vi "Construct Ring Strings Binding.vi"(10 "Ring Refnum":refnum<vi>) -> (0 "error out":errorcluster, 3 "RingStringsBinding":refnum<class "RingStringsBinding.lvclass">)   [LabVIEW 2019, in "RingStringsBinding.lvclass"]
doc: "<License>\nCopyright © 2017 Composed Systems, LLC | All rights reserved\nwww.composed.io\n\nAuthor: Ethan Stern <ethan.stern@composed.io>\n\nThis software is provided \"AS IS\" WITHOUT WARRANTIES, either express or implied, AND IS FOR EDUCATIONAL PURPOSES ONLY.\n</License>MVA Framework 1.0.4.16\nEthan Stern - Composed Systems\nCopyright (c) 2017, Composed Systems"
uses:
  <vilib>/gpm_packages/@cs/transport/Source/Concrete/RingStringsBinding/RingStringsBinding.lvclass
  <vilib>/gpm_packages/@cs/transport/Source/Concrete/RingStringsBinding/RingStringsBinding.lvclass/RingStringsBinding.ctl
  <vilib>/Utility/error.llb/Error Cluster From Error Code.vi
  <vilib>/ErrorRing/Error Ring.xnode
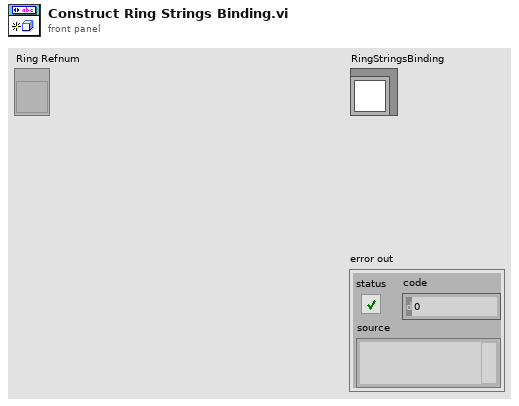
[diagram p1: front panel]
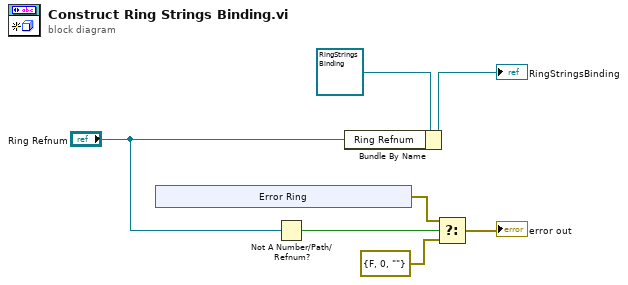
[diagram p0: block diagram]
diagram:
  n1 = xnode "Error Ring"() -> ("error out"=w4:errorcluster)
  n2 = Not A Number/Path/Refnum?(number/path/refnum="Ring Refnum") -> (NaN/Path/Refnum?=w1:bool)
  n3 = Bundle By Name(cluster=refnum<class "RingStringsBinding.lvclass"> refnum ("NamedNumericStringsBinding"), "Ring Refnum"="Ring Refnum") -> (→"RingStringsBinding":refnum<class "RingStringsBinding.lvclass">)
  n4 = Select(t=w4, s=w1, f=errorcluster {"status"=FALSE, "code"=0, "source"=""} ("error constant")) -> (s? t:f=→"error out":errorcluster)
